vi "xlxsOpen.vi"(0 "PIP Instruction Path":path=path "C:/specsheetsConsole/Sheets/ConsoleProcedures.xlsx", 5 "Sheet#":i32, 11 "error in (no error)":errorcluster) -> (4 "Shared_strings":string[][](array[string]), 6 "Sheet_name":string, 8 "Shared_strings 2":string[][](array[string]), 10 "Sheet_name 2":string, 15 "error out":errorcluster)   [LabVIEW 2018]
uses:
  <vilib>/ATEsystem/CLAUDIE_xlsx/Excel_class/Read_excel/Open xlsx.vi
  <vilib>/ATEsystem/CLAUDIE_xlsx/Excel_class/Excel_class.lvclass
panel:
  in  "Sheet# 2":i32=3
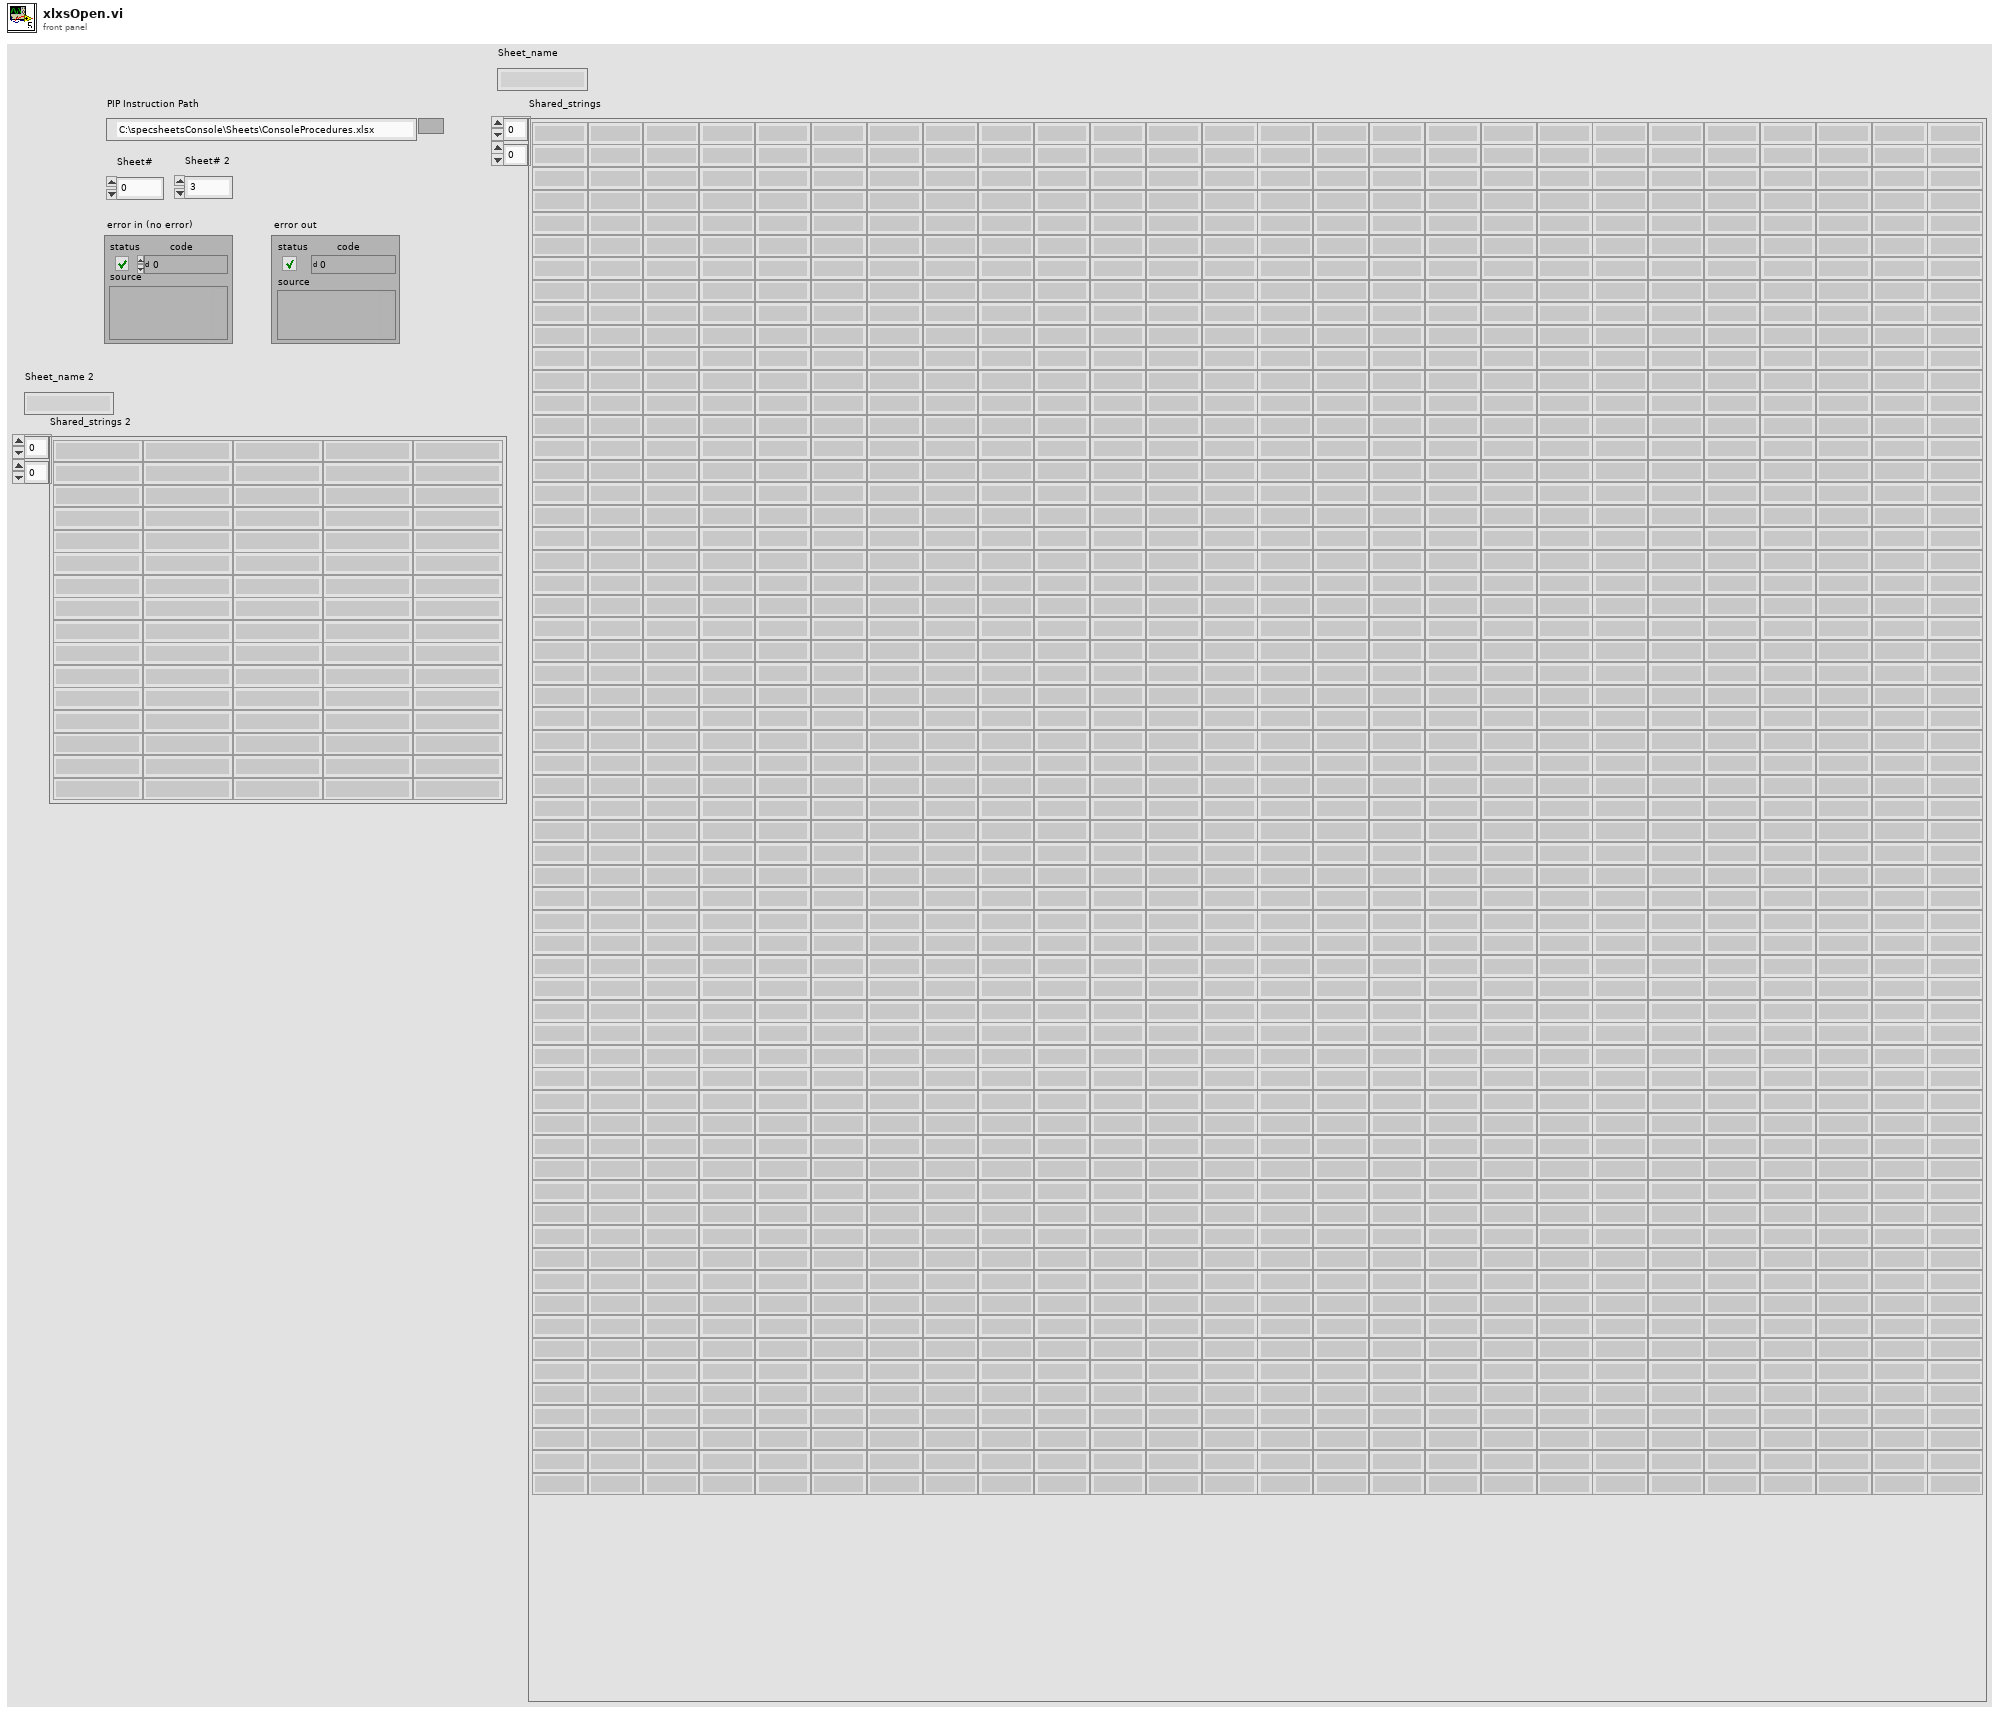
[diagram p1: front panel]
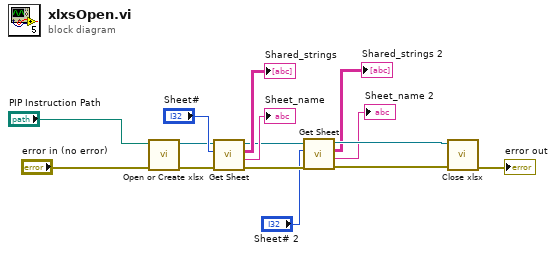
[diagram p0: block diagram]
diagram:
  n1 = call-poly <vilib>:"Open or Create xlsx.vi"("error in (no error)"="error in (no error)", "File Path"="PIP Instruction Path") -> ("error out"=w12:errorcluster, "Excel_class"=w11:refnum<class "Excel_class.lvclass">)  [unwired: 8 in]
  n2 = call <vilib>:"Get Sheet.vi"("error in (no error)"=w12, "List_index"="Sheet#", "Excel_class"=w11) -> ("error out"=w6:errorcluster, "Sheet_name"=→"Sheet_name":string, "Shared_strings"=→"Shared_strings":string[][], "Excel_class"=w7:refnum<class "Excel_class.lvclass">)  [unwired: 5 in]
  n3 = call <vilib>:"Get Sheet.vi"("error in (no error)"=w6, "List_index"="Sheet# 2", "Excel_class"=w7) -> ("error out"=w4:errorcluster, "Sheet_name"=→"Sheet_name 2":string, "Shared_strings"=→"Shared_strings 2":string[][], "Excel_class"=w3:refnum<class "Excel_class.lvclass">)  [unwired: 5 in]
  n4 = call <vilib>:"Close xlsx.vi"("error in (no error)"=w4, "Excel_class"=w3) -> ("error out"=→"error out":errorcluster)  [unwired: 9 in]
